vi "IHM_GetRef.vi"(8 "Error In":errorcluster caption="Entrée d'erreur", 11 "CtrlName":string) -> (0 "Error Out":errorcluster caption="Sortie d'erreur", 1 "Class":string, 2 "Ref":refnum<vi>, 3 "CtrlRef":T1)   [LabVIEW 2013]
uses:
  CTL/CtrlRef.ctl
  FGV/STANDARD/Action.ctl
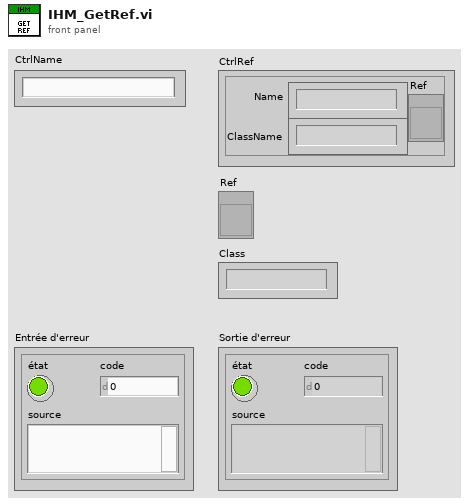
[diagram p1: front panel]
types:
  T1 = typedef "CtrlRef.ctl" = cluster{"Name":string, "Ref":refnum<vi>, "ClassName":string}
  T2 = typedef "Action.ctl" = enum16{"SET", "GET"}
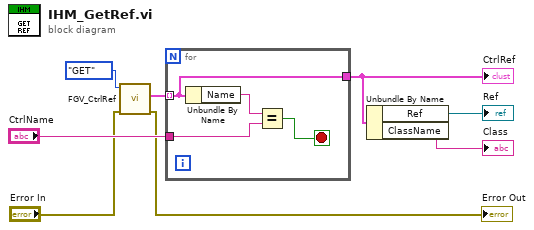
[diagram p0: block diagram]
diagram:
  n1 = call "FGV_CtrlRef.vi"("error in (no error)"="Error In", "Action"=Action."GET") -> ("error out"=→"Error Out":errorcluster, "CtrlsRefs_OUT"=w6:T1[])  [unwired: 8 in]
  n2 = for {
    tunnel: w6 -> [w10] mode=indexing
    tunnel: "CtrlName" -> [w12]
    tunnel: [w10] -> w3
    stop <- w9 stop-if-true
    n3 = Unbundle By Name(w10) -> ("Name"=w11:string)
    n4 = Equal?(x=w11, y=w12) -> (x = y?=w9:bool)
  }
  "CtrlRef" <- w3
  n5 = Unbundle By Name(w3) -> ("Ref"=→"Ref":refnum<vi>, "ClassName"=→"Class":string)
